vi "Channel Probe.vi"(2 "channelOp":enum16{"init", "write", "read", "probe"}(ring)=enum."write", 3 "tagData in":refnum<class "TagData.lvclass">) -> (1 "tagData out":refnum<class "TagData.lvclass">)   [LabVIEW 2020, in "Tag-a[.](c(a[.](stamp),a[.](dbl))).lvlib"]
doc: "Displays the status of the channel as the channel is modified by the various endpoints and gives the user ways to pause the application using the channel."
uses:
  <extravilib>/ChannelInstances/Tag-a[.](c(a[.](stamp),a[.](dbl))).lvlib
  <extravilib>/ChannelInstances/Tag-a[.](c(a[.](stamp),a[.](dbl)))/TagData.lvclass
panel:
  in  "Single Step":bool
  out "Tag Name":string="<Unnamed>"
  in  "Sequence Number To Match":i32
  in  "Pause when Sequence Number matches":bool
  in  "Value To Match":cluster{timestamp[], dbl[]}[](array[cluster])
  in  "Pause when Tag Value matches":bool
  in  "Pause when aborted":bool
  in  "Step To Next Write":bool
  in  "Play":bool
  out "Aborted?":bool
  out "Sequence Number":i32
  out "Tag Name":string
  out "Tag Value":cluster{timestamp[], dbl[]}[](array[cluster])
  in  "Pause":bool
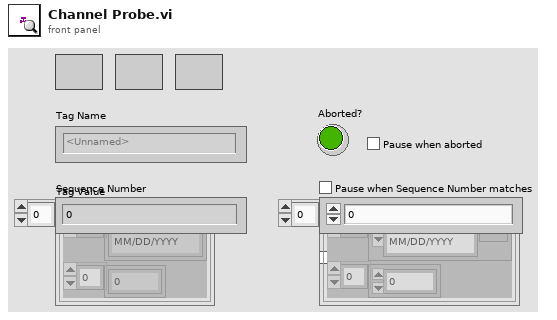
[diagram p1: front panel]
types:
  T1 = enum32{"Invalid", "Standard", "Closed", "Hidden", "Minimized", "Maximized"}
  T2 = typedef "LVPointTypeDef.ctl" = cluster{"Horizontal":i16, "Vertical":i16}
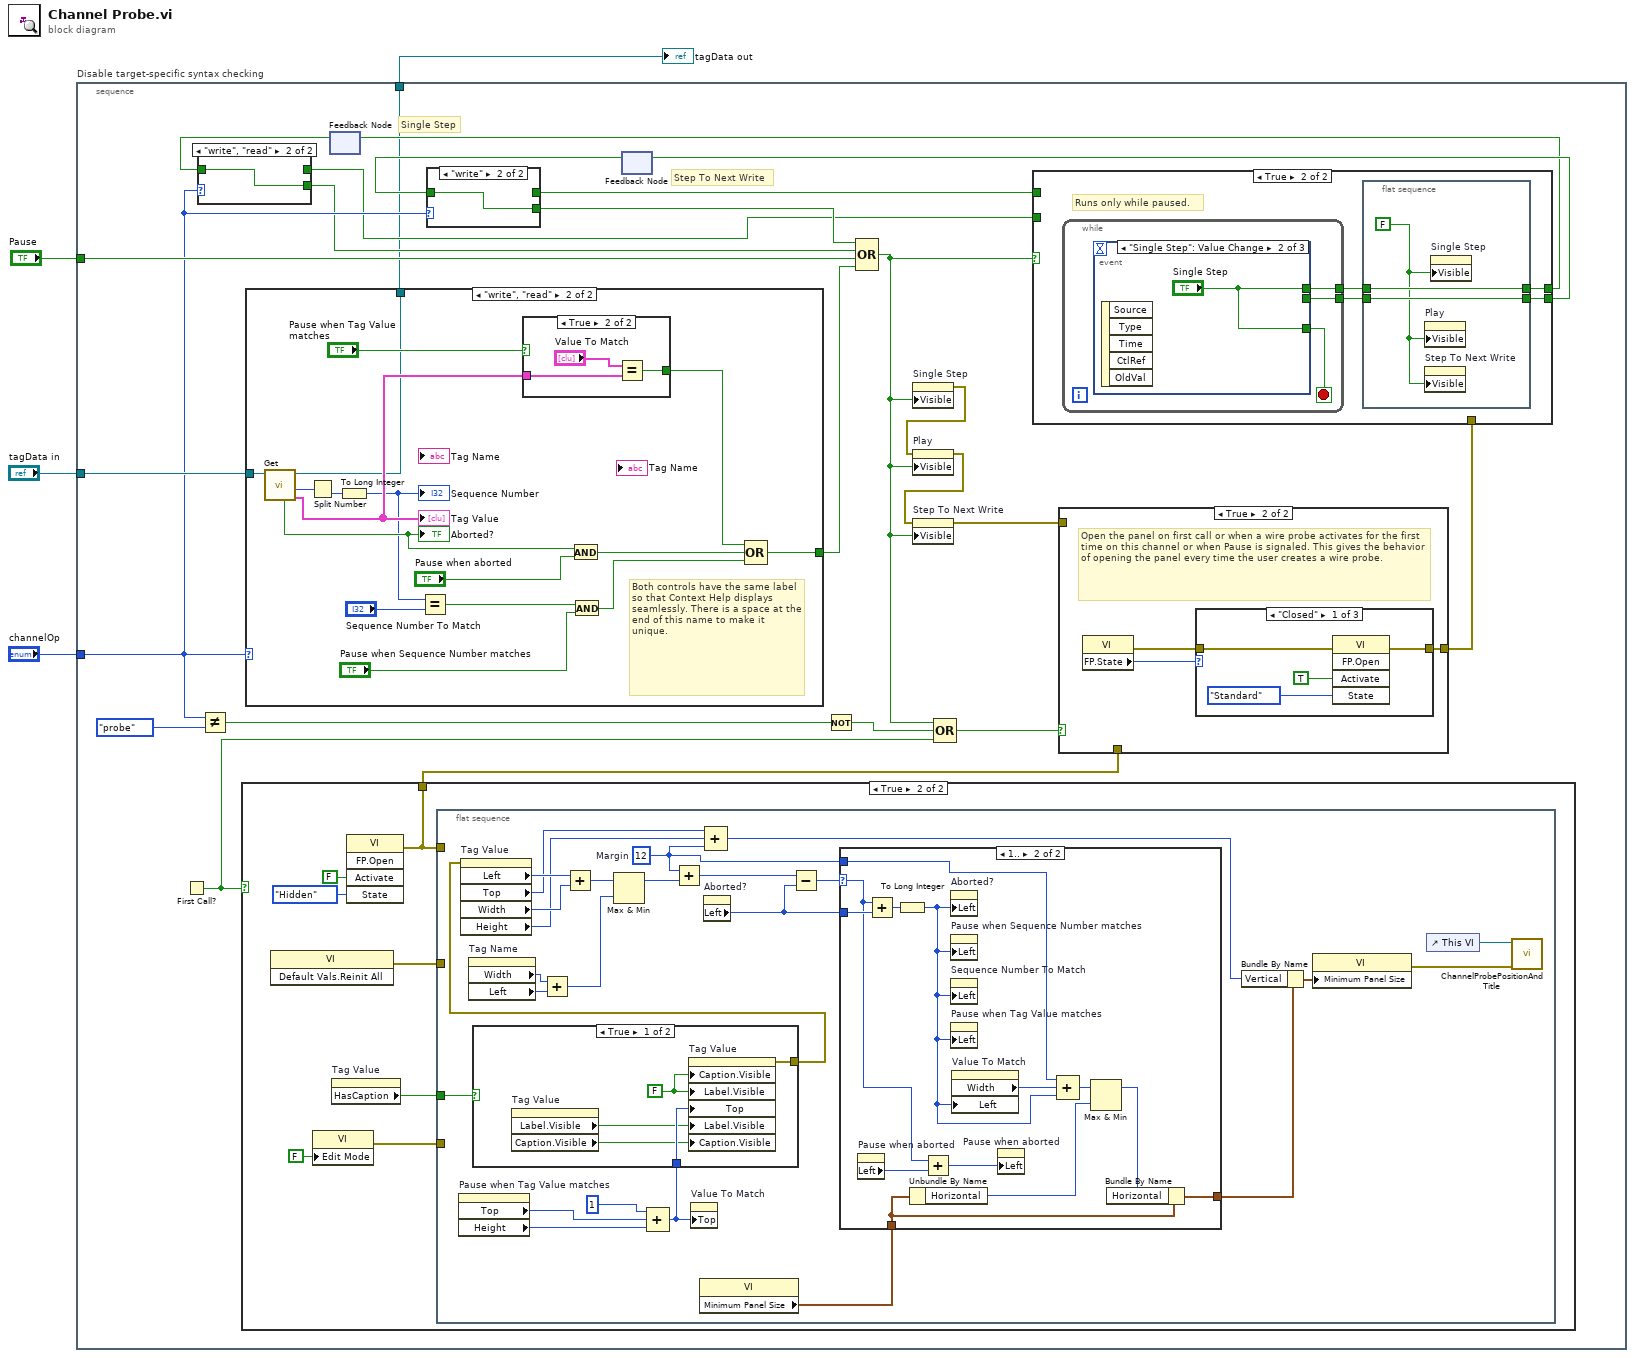
[diagram p0: block diagram]
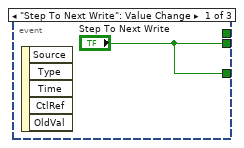
[diagram p5: hidden frame]
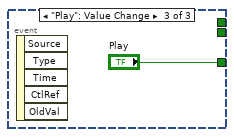
[diagram p6: hidden frame]
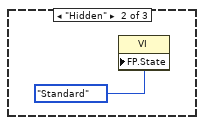
[diagram p10: hidden frame]
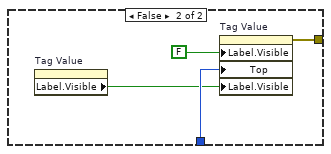
[diagram p13: hidden frame]
diagram:
  n1 = stacked-sequence "Disable target-specific syntax checking" {
    tunnel: "tagData in" -> [w28]
    tunnel: "Pause" -> [w21]
    tunnel: "channelOp" -> [w11]
    tunnel: [w5] -> w1
    frame #0 {
      # "Step To Next Write"
      # "Single Step"
      n2 = First Call?() -> (First Call?: T/F=w26:bool)
      n3 = Not Equal?(x=w11, y=enum16{"init", "write", "read", "probe"}."probe" ("channelOp 2")) -> (x != y?=w23:bool)
      n4 = case shown="True" w26 {
        tunnel: [_ w77] -> w14
        frame False {
        }
        frame True {
          n5 = invoke class="VI" method="Default Vals.Reinit All"() -> (error out=w78:errorcluster)  [unwired: 3 in, 2 out]
          n6 = property class="VI"("Edit Mode"=FALSE ("Edit Mode On Open")) -> (error out=w79:errorcluster)  [unwired: 2 in, 1 out]
          n7 = property on="Tag Value" class="Arr (strict)"() -> ("HasCaption"=w76:bool)  [unwired: 2 in, 2 out]
          n8 = invoke class="VI" method="FP.Open"("Activate"=FALSE ("Activate?"), "State"=T1."Hidden") -> (error out=w77:errorcluster)  [unwired: 3 in, 4 out]
          n9 = flat-sequence {
            tunnel: w77 -> [_]
            tunnel: w79 -> [_]
            tunnel: w78 -> [_]
            tunnel: w76 -> [w91]
            frame #0 {
              w89 = 12  # Margin
              n10 = property on="Pause when Tag Value matches" class="Bool (strict)"() -> ("Top"=w99:i32, "Height"=w98:u32)  [unwired: 2 in, 2 out]
              n11 = property on="Tag Name" class="Str"() -> ("Width"=w87:u32, "Left"=w86:i32)  [unwired: 2 in, 2 out]
              n12 = Add(x=w87, y=w86) -> (x+y=w84:u32)
              n13 = Compound Arithmetic op=ADD(u32 1 ("value"), w99, w98) -> (w97:u32)
              n14 = case shown="True" w91 {
                tunnel: w97 -> [w112 w116]
                tunnel: [w111 w115] -> w95
                frame True {
                  w108 = FALSE ("Label.Visible")
                  n15 = property on="Tag Value" class="Arr (strict)"() -> ("Label.Visible"=w110:bool, "Caption.Visible"=w109:bool)  [unwired: 2 in, 2 out]
                  n16 = property on="Tag Value" class="Arr (strict)"("Caption.Visible"=w108, "Label.Visible"=w108, "Top"=w112, "Label.Visible"=w110, "Caption.Visible"=w109) -> (error out=w111:errorcluster)  [unwired: 2 in, 1 out]
                }
                frame False {
                  n17 = property on="Tag Value" class="Arr (strict)"() -> ("Label.Visible"=w113:bool)  [unwired: 2 in, 2 out]
                  n18 = property on="Tag Value" class="Arr (strict)"("Label.Visible"=FALSE, "Top"=w116, "Label.Visible"=w113) -> (error out=w115:errorcluster)  [unwired: 2 in, 1 out]
                }
              }
              n19 = property on="Tag Value" class="Arr (strict)"(error in=w95) -> ("Left"=w107:i32, "Top"=w102:i32, "Width"=w106:u32, "Height"=w101:u32)  [unwired: 1 in, 2 out]
              n20 = Add(x=w107, y=w106) -> (x+y=w85:u32)
              n21 = Max & Min(x=w85, y=w84) -> (max(x,y)=w83:u32)  [unwired: 1 out]
              n22 = Add(x=w89, y=w83) -> (x+y=w105:u32)
              n23 = property on="Value To Match" class="Arr (strict)"("Top"=w97) -> ()  [unwired: 2 in, 2 out]
              n24 = property class="VI"() -> ("Minimum Panel Size"=w90:T2)  [unwired: 2 in, 2 out]
              n25 = property on="Aborted?" class="Bool (strict)"() -> ("Left"=w103:i32)  [unwired: 2 in, 2 out]
              n26 = Compound Arithmetic op=ADD(w102, w101, w89) -> (w100:u32)
              n27 = Subtract(x=w105, y=w103) -> (x-y=w104:u32)
              n28 = case shown="1.." w104 {
                selector: w104 -> [_ w128]
                tunnel: w103 -> [_ w130]
                tunnel: w90 -> [w117 w120]
                tunnel: w89 -> [_ w123]
                tunnel: [w117 w118] -> w88
                frame Default {
                }
                frame 1.. {
                  n29 = property on="Pause when aborted" class="Bool (strict)"() -> ("Left"=w129:i32)  [unwired: 2 in, 2 out]
                  n30 = Add(x=w128, y=w130) -> (x+y=w126:u32)
                  n31 = To Long Integer(number=w126) -> (32bit integer=w124:i32)
                  n32 = Unbundle By Name(w120) -> ("Horizontal"=w121:i16)
                  n33 = Add(x=w128, y=w129) -> (x+y=w127:u32)
                  n34 = property on="Aborted?" class="Bool (strict)"("Left"=w124) -> ()  [unwired: 2 in, 2 out]
                  n35 = property on="Pause when Sequence Number matches" class="Bool (strict)"("Left"=w124) -> ()  [unwired: 2 in, 2 out]
                  n36 = property on="Sequence Number To Match" class="DigNum (strict)"("Left"=w124) -> ()  [unwired: 2 in, 2 out]
                  n37 = property on="Pause when Tag Value matches" class="Bool (strict)"("Left"=w124) -> ()  [unwired: 2 in, 2 out]
                  n38 = property on="Value To Match" class="Arr (strict)"("Left"=w124) -> ("Width"=w125:u32)  [unwired: 2 in, 2 out]
                  n39 = property on="Pause when aborted" class="Bool (strict)"("Left"=w127) -> ()  [unwired: 2 in, 2 out]
                  n40 = Compound Arithmetic op=ADD(w123, w125, w124) -> (w122:u32)
                  n41 = Max & Min(x=w122, y=w121) -> (max(x,y)=w119:u32)  [unwired: 1 out]
                  n42 = Bundle By Name(cluster=w120, "Horizontal"=w119) -> (w118:T2)
                }
              }
              n43 = Bundle By Name(cluster=w88, "Vertical"=w100) -> (w94:T2)
              n44 = property class="VI"("Minimum Panel Size"=w94) -> (error out=w93:errorcluster)  [unwired: 2 in, 1 out]
              n45 = control-ref of="This VI"() -> (w92:refnum<vi>)
              n46 = call <resource>:"ChannelProbePositionAndTitle.vi"("error in (no error)"=w93, "VI in"=w92) -> ()  [unwired: 8 in, 2 out]
            }
          }
        }
      }
      n47 = case shown="\"write\", \"read\"" w11 {
        tunnel: w28 -> [w48 w64]
        tunnel: [_ w53] -> w22
        tunnel: [w48 w51] -> w5
        frame Default {
        }
        frame "write", "read" {
          # "Both controls have the same label so that Context Help displays seamlessly. There is a space at the end of this name to make it unique."
          n48 = call <extravilib>:"Get.vi"("TagData in"=w64) -> ("element"=w55:cluster{timestamp[], dbl[]}[], "sequence"=w52:u64, "TagData out"=w51:refnum<class "TagData.lvclass">, "aborted?"=w61:bool)  [unwired: 6 in, 1 out]
          "Tag Value" <- w55
          "Aborted?" <- w61
          n49 = Split Number(x=w52) -> (lo(x)=w50:u32)  [unwired: 1 out]
          n50 = To Long Integer(number=w50) -> (32bit integer=w49:i32)
          "Sequence Number" <- w49
          n51 = Equal?(x=w49, y="Sequence Number To Match") -> (x = y?=w59:bool)
          n52 = case shown="True" "Pause when Tag Value matches" {
            tunnel: w55 -> [_ w66]
            tunnel: [_ w65] -> w54
            frame False {
            }
            frame True {
              n53 = Equal?(x="Value To Match", y=w66) -> (x = y?=w65:bool)
            }
          }
          n54 = And(x=w61, y="Pause when aborted") -> (x .and. y?=w60:bool)
          n55 = And(x=w59, y="Pause when Sequence Number matches") -> (x .and. y?=w57:bool)
          n56 = Compound Arithmetic op=OR(w54, w60, w57) -> (w53:bool)
        }
      }
      n57 = feedback #1() -> (w12:bool)  [unwired: 1 in]
      n58 = case shown="\"write\", \"read\"" w11 {
        tunnel: w12 -> [w29 w30]
        tunnel: [_ w30] -> w9
        tunnel: [w29 _] -> w8
        frame Default {
        }
        frame "write", "read" {
        }
      }
      n59 = feedback #2() -> (w19:bool)  [unwired: 1 in]
      n60 = case shown="\"write\"" w11 {
        tunnel: w19 -> [w31 w32]
        tunnel: [_ w32] -> w10
        tunnel: [w31 _] -> w18
        frame Default {
        }
        frame "write" {
        }
      }
      n61 = Not(x=w23) -> (.not. x?=w27:bool)
      n62 = Compound Arithmetic op=OR(w10, w9, w21, w22) -> (w7:bool)
      n63 = property on="Single Step" class="Bool"("Visible"=w7) -> (error out=w6:errorcluster)  [unwired: 2 in, 1 out]
      n64 = property on="Play" class="Bool"(error in=w6, "Visible"=w7) -> (error out=w17:errorcluster)  [unwired: 1 in, 1 out]
      n65 = property on="Step To Next Write" class="Bool"(error in=w17, "Visible"=w7) -> (error out=w16:errorcluster)  [unwired: 1 in, 1 out]
      n66 = Compound Arithmetic op=OR(w7, w27, w26) -> (w25:bool)
      n67 = case shown="True" w25 {
        tunnel: w16 -> [_ _]
        tunnel: [_ w68] -> w15
        tunnel: w14 -> [_ _]
        frame False {
        }
        frame True {
          # "Open the panel on first call or when a wire probe activates for the first time on this channel or when Pause is signaled. This gives the behavior of opening the panel every time the user creates a wire probe."
          n68 = property class="VI"() -> (error out=w69:errorcluster, "FP.State"=w70:T1)  [unwired: 2 in, 1 out]
          n69 = case shown="\"Closed\"" w70 {
            tunnel: w69 -> [w74 _ _]
            tunnel: [w71 _ _] -> w68
            frame "Closed" {
              n70 = invoke class="VI" method="FP.Open"(error in=w74, "Activate"=TRUE ("Activate?"), "State"=T1."Standard") -> (error out=w71:errorcluster)  [unwired: 2 in, 4 out]
            }
            frame "Hidden" {
              n71 = property class="VI"("FP.State"=T1."Standard" ("Front Panel Window:State")) -> ()  [unwired: 2 in, 2 out]
            }
            frame Default {
            }
          }
        }
      }
      n72 = case shown="True" w7 {
        tunnel: [w34 w38] -> w20
        tunnel: w18 -> [w34 _]
        tunnel: w15 -> [_ _]
        tunnel: [w33 w36] -> w13
        tunnel: w8 -> [w33 _]
        frame False {
        }
        frame True {
          # "Runs only while paused."
          n73 = while {
            tunnel: [w44] -> w37
            tunnel: [w42] -> w35
            stop <- w43 stop-if-true
            n74 = event shown="[1] \"Single Step\": Value Change" {
              selector: _ -> [_ _ _]
              dyn-events: _ -> [_ _ _]
              timeout: _ -> [_ _ _]
              tunnel: ["Step To Next Write" _ _] -> w44
              tunnel: ["Step To Next Write" "Single Step" "Play"] -> w43
              tunnel: [_ "Single Step" _] -> w42
              event "Step To Next Write": Value Change {
                n75 = event-data() -> ()  [unwired: 1 in, 5 out]
              }
              event "Single Step": Value Change {
                n76 = event-data() -> ()  [unwired: 1 in, 5 out]
              }
              event "Play": Value Change {
                n77 = event-data() -> ()  [unwired: 1 in, 5 out]
              }
            }
          }
          n78 = flat-sequence {
            tunnel: [w41] -> w38
            tunnel: w37 -> [w41]
            tunnel: [w40] -> w36
            tunnel: w35 -> [w40]
            frame #0 {
              w39 = FALSE ("Pause")
              n79 = property on="Play" class="Bool"("Visible"=w39) -> ()  [unwired: 2 in, 2 out]
              n80 = property on="Step To Next Write" class="Bool"("Visible"=w39) -> ()  [unwired: 2 in, 2 out]
              n81 = property on="Single Step" class="Bool"("Visible"=w39) -> ()  [unwired: 2 in, 2 out]
            }
          }
        }
      }
      n82 = feedback-in #1(w13) -> ()
      n83 = feedback-in #2(w20) -> ()
    }
  }
  "tagData out" <- w1
